vi "Set_APC_Power_dBm.vi"(0 ".NET Reference in":refnum<k24>, 1 "Setting Power":dbl, 3 "error in (no error)":errorcluster) -> (7 "Reference out":refnum<k24>, 10 "error out":errorcluster)   [LabVIEW 2017]
doc: "set Power"
uses:
  D:/test/ILSTS/LV_IL/LV_IL_Sample_x86/DLL/InstrumentDLL.dll
  DLL/InstrumentDLL.dll
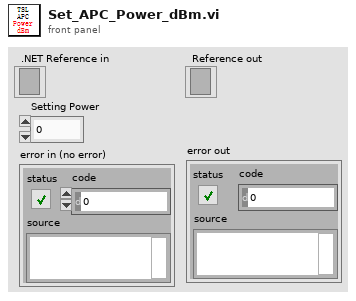
[diagram p1: front panel]
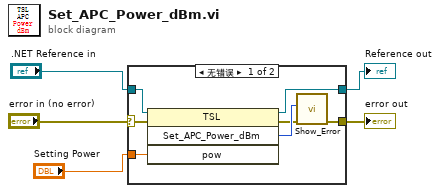
[diagram p0: block diagram]
diagram:
  n1 = case shown="无错误" "error in (no error)" {
    selector: "error in (no error)" -> [w9 w14]
    tunnel: "Setting Power" -> [w12 _]
    tunnel: ".NET Reference in" -> [w11 w13]
    tunnel: [w10 w13] -> w3
    tunnel: [w6 w14] -> w2
    frame No Error {
      n2 = invoke on="调用节点" class="TSL" method="Set_APC_Power_dBm"(reference=w11, error in=w9, "pow"=w12) -> (reference out=w10:refnum<k24>, error out=w7:errorcluster, "Set_APC_Power_dBm"=w8:i32)  [unwired: 1 in, 1 out]
      n3 = call "Show_Error.vi"("error in (no error)"=w7, "Error"=w8) -> ("error out"=w6:errorcluster)  [unwired: 9 in]
    }
    frame Error {
    }
  }
  "Reference out" <- w3
  "error out" <- w2
